vi "RemoveByIndex.vi"(8 "error in (no error)":errorcluster, 10 "Name":i32, 11 "CollectionByRef in":refnum<class "CollectionByRef.lvclass">) -> (0 "error out":errorcluster, 1 "found":bool, 2 "LabVIEW Object Removed":refnum<class>, 3 "CollectionByRef out":refnum<class "CollectionByRef.lvclass">)   [LabVIEW 2021, in "Collection.lvlib" / "CollectionByRef.lvclass"]
uses:
  CollectionByRef.lvclass
  CollectionByRef.lvclass/CollectionByRef.ctl
  CollectionByValue/CollectionByValue.lvclass
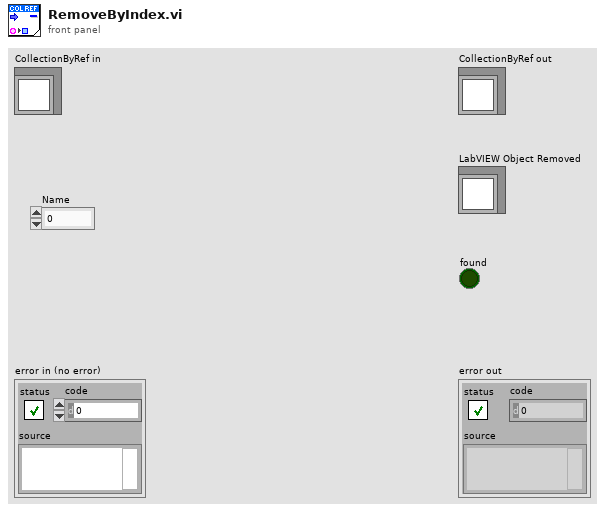
[diagram p1: front panel]
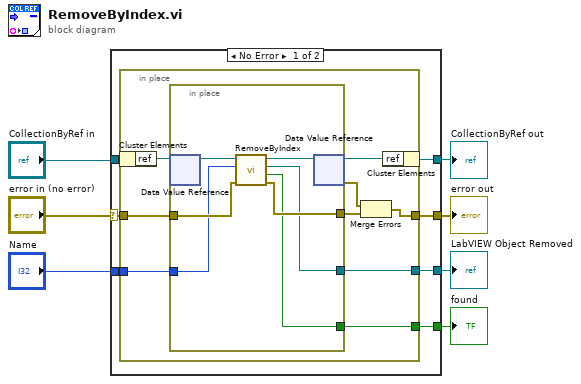
[diagram p0: block diagram]
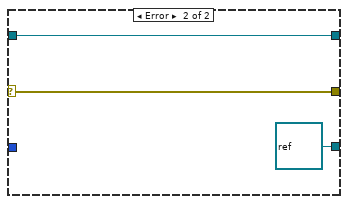
[diagram p2: hidden frame]
diagram:
  n1 = case shown="No Error" "error in (no error)" {
    selector: "error in (no error)" -> [w12 w33]
    tunnel: [w11 w33] -> w5
    tunnel: [w13 w32] -> w6
    tunnel: "CollectionByRef in" -> [w14 w32]
    tunnel: "Name" -> [w10 _]
    tunnel: [w9 refnum<class> refnum ("LabVIEW Object Removed")] -> w2
    tunnel: [w8 _] -> w1
    frame No Error {
      n2 = in-place {
        in-place-border: w12 -> [w21]
        in-place-border: [w18] -> w11
        in-place-border: w10 -> [w17]
        in-place-border: [w16] -> w9
        in-place-border: [w15] -> w8
        n3 = in-place-cluster #1(w14) -> ("ref"=w22:refnum<data-value>)
        n4 = in-place {
          in-place-border: w21 -> [w28]
          in-place-border: [w27] -> w19
          in-place-border: w17 -> [w24]
          in-place-border: [w25] -> w16
          in-place-border: [w26] -> w15
          n5 = in-place-dvr #2(w22) -> (w30:refnum<class "CollectionByValue.lvclass">)  [unwired: 1 out]
          n6 = call "RemoveByIndex.vi"("error in (no error)"=w28, "Index"=w24, "Collection in"=w30) -> ("error out"=w27:errorcluster, "found"=w26:bool, "LabVIEW Object Removed"=w25:refnum<class>, "Collection out"=w29:refnum<class "CollectionByValue.lvclass">)  [unwired: 4 in, 1 out]
          n7 = in-place-dvr #2(w29) -> (w23:refnum<data-value>, w20:errorcluster)
        }
        n8 = Merge Errors(w20, w19) -> (w18:errorcluster)
        n9 = in-place-cluster #1("ref"=w23) -> (w13:refnum<class "CollectionByRef.lvclass">)
      }
    }
    frame Error {
    }
  }
  "error out" <- w5
  "CollectionByRef out" <- w6
  "LabVIEW Object Removed" <- w2
  "found" <- w1
